vi "Slide.vi"(8 "error in (no error)":errorcluster, 9 "Action":T1, 10 "CtlRef":refnum<vi>, 11 "SlideEngine.lvclass":refnum<class "SlideEngine.lvclass">) -> (0 "error out":errorcluster, 3 "SlideEngine.lvclass Out":refnum<class "SlideEngine.lvclass">)   [LabVIEW 2012, in "SlideEngine.lvclass"]
doc: "Use this VI to queue a sliding action for a particular control."
uses:
  SlideEngine.lvclass
  SlideActions.ctl
  SlideEngine.lvclass/SlideEngine.ctl
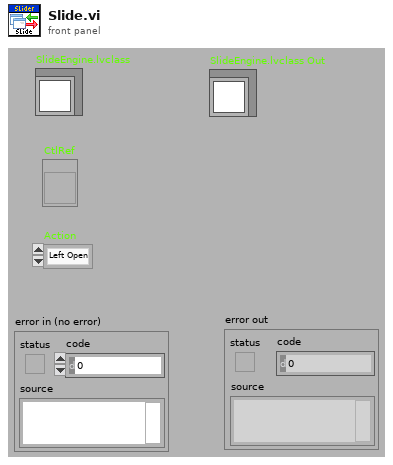
[diagram p1: front panel]
types:
  T1 = typedef "SlideActions.ctl" = enum16{"Left Open", "Left Close"}
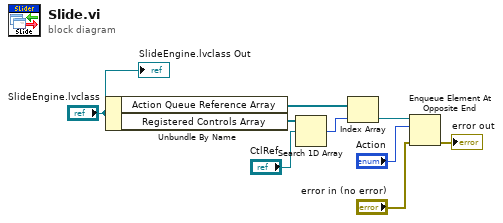
[diagram p0: block diagram]
diagram:
  n1 = Unbundle By Name("SlideEngine.lvclass") -> ("Action Queue Reference Array"=w7:refnum<queue>[], "Registered Controls Array"=w9:refnum<vi>[])
  n2 = Search 1D Array(1D array=w9, element="CtlRef") -> (index of element=w8:i32)  [unwired: 1 out]
  n3 = Index Array(array=w7, index=w8) -> (element=w6:refnum<queue>)
  n4 = Enqueue Element At Opposite End(queue=w6, element="Action", error in (no error)="error in (no error)") -> (error out=→"error out":errorcluster)  [unwired: 3 out]
  "SlideEngine.lvclass Out" <- "SlideEngine.lvclass"
